vi "Netburner_cntlfull.vi"(0 "Phase Volt":dbl=6.500000000000002 min=-9.0 max=9.0 step=0.0005 format="%_5f", 1 "Tune Volt":dbl=0.3670000000000009 min=-9.9 max=9.9 step=0.0005 format="%_5g", 3 "# Data":i32=80 min=1 max=500 step=1, 5 "IF Atten (dB)":i8=3 min=0 max=31 step=1, 7 "NMR ADC":i32 min=0 max=3 step=1, 8 "Hi Gain":bool, 9 "Tank RF":bool, 11 "LogOff Volt":dbl=-5.996000000000003 min=0.0 max=9.0 step=0.0005 format="%_5f", 12 "IFOff Volt":dbl=5.450461000000012 min=-9.9 max=9.9 step=0.0005 format="%_4g", 14 "# f steps":i32=81 min=1 max=1000 step=1) -> (2 "Temp (C)":dbl=26.88 format="%#_5g", 4 "ADC value":dbl[](array[numeric])=[-0.0314, -0.0313, -0.0297, -0.0295, -0.0285, -0.0272, -0.026, -0.0257, -0.0236, -0.0229, -0.0227, -0.0232, -0.0213, -0.0193, -0.0187, -0.018, -0.0166, -0.0148, -0.0136, -0.0136, -0.0124, -0.0123, -0.0121, -0.0127, -0.0131, -0.0123, -0.0127, -0.0125, -0.0133, -0.0128, -0.0117, -0.012, -0.0128, -0.0138, -0.0149, -0.0166, -0.0211, -0.0291, -0.0424, -0.043, -0.0352, -0.0325, -0.0302, -0.0273, -0.0269, -0.0277, -0.026, -0.0263, -0.0242, -0.021, -0.0178, -0.0171, -0.0172, -0.0168, -0.0161, -0.0168, -0.0178, -0.0197, -0.0204, -0.0197, -0.0175, -0.0187, -0.0188, -0.0202, -0.0207, -0.0229, -0.0238, -0.0251, -0.0264, -0.0268, -0.0278, -0.0301, -0.0313, -0.0334, -0.0364, -0.0377, -0.0382, -0.0394, -0.043, -0.0442, -0.0438], 6 "ADC Std Dev":dbl=0.0009679012345679012 format="%#_4g", 10 "Max ADC":dbl=-0.0117 format="%#_5g", 13 "Volts":dbl=3.245 format="%#_5g", 15 "Min ADC":dbl=-0.0442 format="%#_5g")   [LabVIEW 2013]
uses:
  Global 2.vi
  <vilib>/Analysis/NI_AALBase.lvlib
panel:
  in  "First":bool=TRUE
  out "Begin string":string
  out "ADC Voltage Chart":dbl(graph)=-0.0438
  out "Mean ADC":dbl=-0.023260493827160496 format="%#_5g"
  out "ADC result string":string=" 6.5000  0.3670 -5.9960  5.4505 0 80 81 6 0 0\r26.88  3.245  \r\n-0.0314 0.0005  \r\n-0.0313 0.0007  \r\n-0.0297 0.0008  \r\n-0.0295 0.0007  \r\n-0.0285 0.0009  \r\n-0.0272 0.0007  \r\n-0.0260 0.0009  \r\n-0.0257 0.0007  \r\n-0.0236 0.0008  \r\n-0.0229 0.0008  \r\n-0.0227 0.0009  \r\n-0.0232 0.0011  \r\n-0.0213 0.0010  \r\n-0.0193 0.0014  \r\n-0.0187 0.0009  \r\n-0.0180 0.0007  \r\n-0.0166 0.0010  \r\n-0.0148 0.0006  \r\n-0.0136 0.0007  \r\n-0.0136 0.0010  \r\n-0.0124 0.0006  \r\n-0.0123 0.0007  \r\n-0.0121 0.0007  \r\n-0.0127 0.0006  \r\n-0.0131 0.0006  \r\n-0.0123 0.0007  \r\n-0.0127 0.0007  \r\n-0.0125 0.0006  \r\n-0.0133 0.0006  \r\n-0.0128 0.0009  \r\n-0.0117 0.0006  \r\n-0.0120 0.0008  \r\n-0.0128 0.0006  \r\n-0.0138 0.0007  \r\n-0.0149 0.0009  \r\n-0.0166 0.0016  \r\n-0.0211 0.0031  \r\n-0.0291 0.0059  \r\n-0.0424 0.0009  \r\n-0.0430 0.0037  \r\n-0.0352 0.0010  \r\n-0.0325 0.0013  \r\n-0.0302 0.0016  \r\n-0.0273 0.0006  \r\n-0.0269 0.0007  \r\n-0.0277 0.0007  \r\n-0.0260 0.0009  \r\n-0.0263 0.0015  \r\n-0.0242 0.0014  \r\n-0.0210 0.0013  \r\n-0.0178 0.0010  \r\n-0.0171 0.0007  \r\n-0.0172 0.0007  \r\n-0.0168 0.0007  \r\n-0.0161 0.0006  \r\n-0.0168 0.0005  \r\n-0.0178 0.0010  \r\n-0.0197 0.0008  \r\n-0.0204 0.0010  \r\n-0.0197 0.0006  \r\n-0.0175 0.0006  \r\n-0.0187 0.0006  \r\n-0.0188 0.0010  \r\n-0.0202 0.0007  \r\n-0.0207 0.0006  \r\n-0.0229 0.0008  \r\n-0.0238 0.0009  \r\n-0.0251 0.0009  \r\n-0.0264 0.0008  \r\n-0.0268 0.0009  \r\n-0.0278 0.0008  \r\n-0.0301 0.0007  \r\n-0.0313 0.0006  \r\n-0.0334 0.0012  \r\n-0.0364 0.0009  \r\n-0.0377 0.0006  \r\n-0.0382 0.0007  \r\n-0.0394 0.0013  \r\n-0.0430 0.0012  \r\n-0.0442 0.0008  \r\n-0.0438 0.0009  \r\n?\r\n"
  out "#  Data Bytes Read":u32=1523
  out "DAC, ADC String":string=" 6.5000  0.3670 -5.9960  5.4505 0 80 81 6 0 0"
  out "Error Out":errorcluster={"status"=FALSE, "code"=1073676294, "source"="VISA Read in Netburner_RD.vi->Netburner_cntl6.vi"}
  in  "Error In (none)":errorcluster
  out "COM Port #":refnum<visa-resource-name>="COM9"
  # "Netburner ADC/DAC Test Interface"
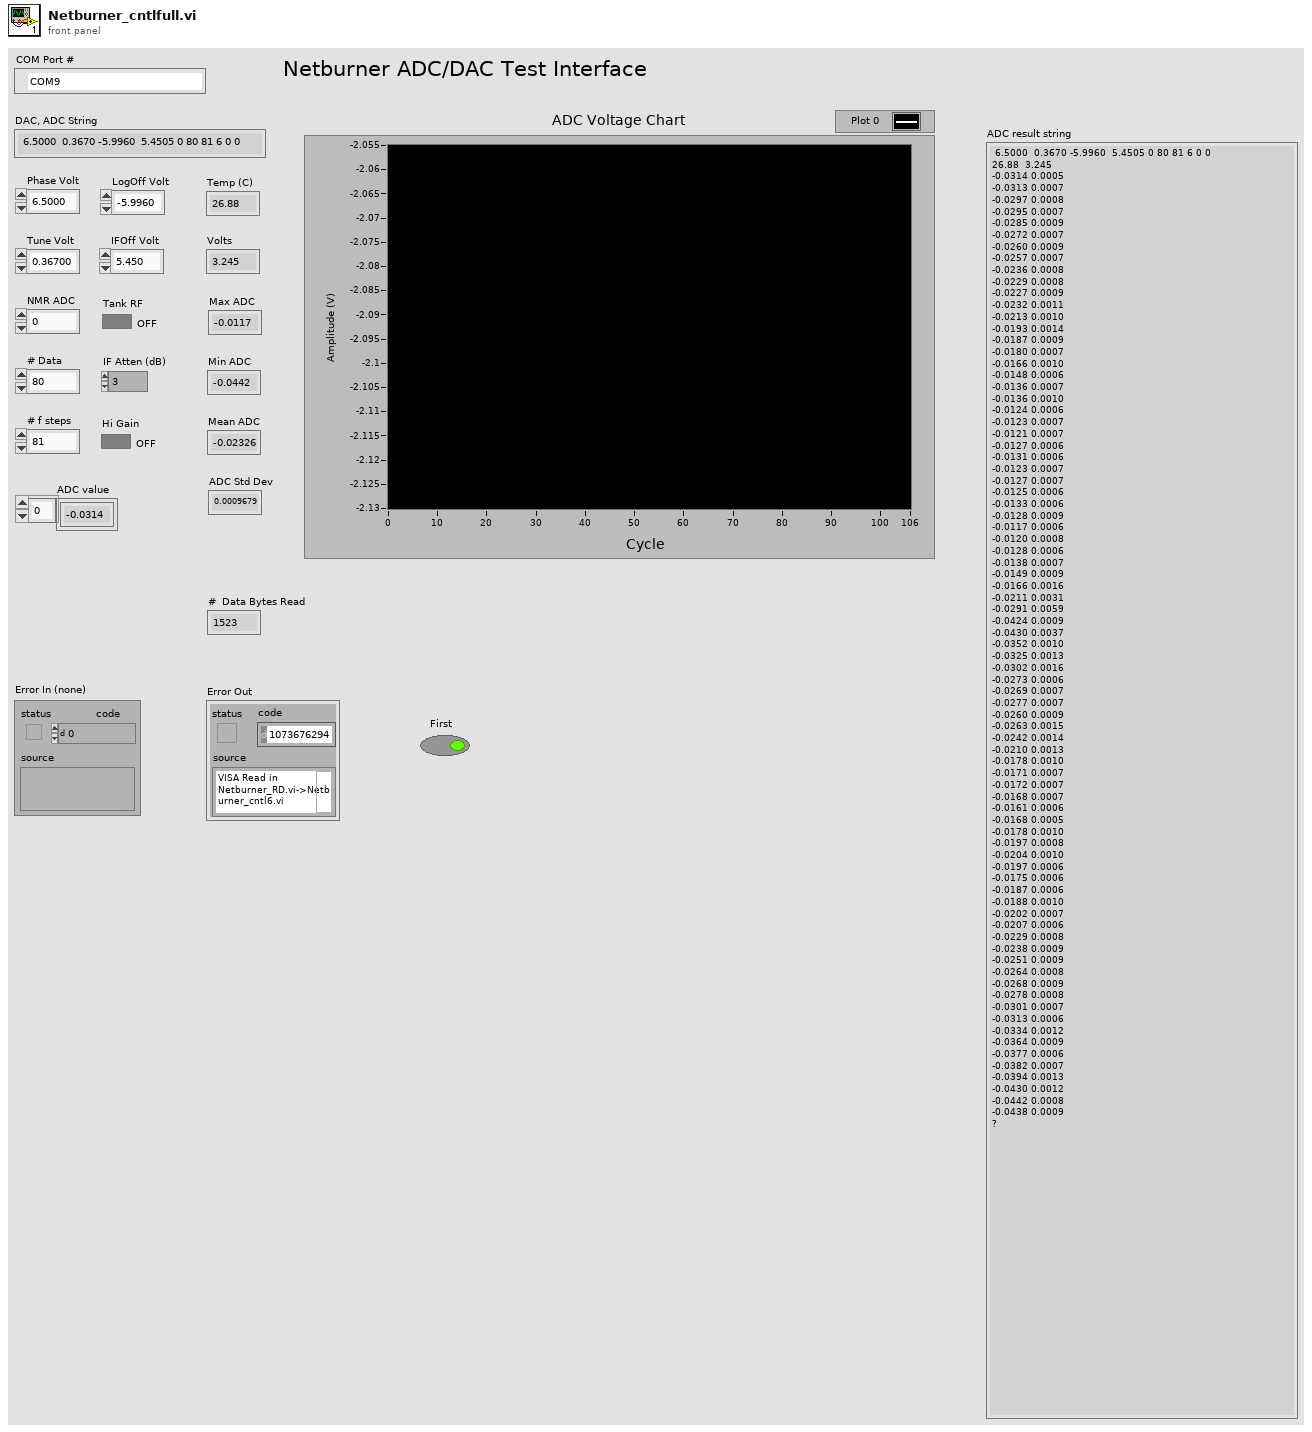
[diagram p1: front panel]
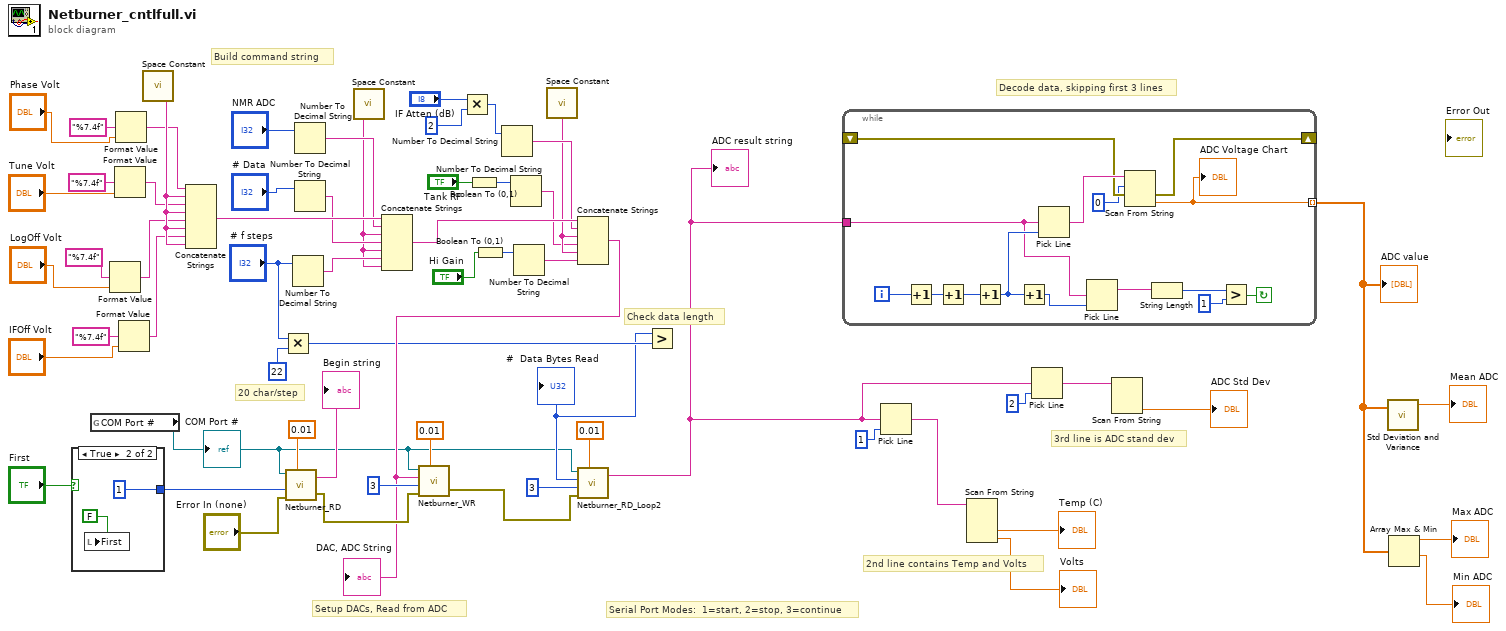
[diagram p0: block diagram]
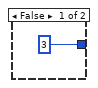
[diagram p2: hidden frame]
diagram:
  # "3rd line is ADC stand dev"
  # "20 char/step"
  # "Check data length"
  # "2nd line contains Temp and Volts"
  # "Build command string"
  # "Decode data, skipping first 3 lines"
  # "Serial Port Modes:  1=start, 2=stop, 3=continue"
  # "Setup DACs, Read from ADC"
  n1 = case shown="True" "First" {
    tunnel: [3 1] -> w6
    frame False {
    }
    frame True {
      n2 = local write "First"(FALSE) -> ()
    }
  }
  n3 = global read "Global 2.vi" "COM Port #"() -> (w5:refnum<visa-resource-name>)
  "COM Port #" <- w5
  n4 = Format Value(format string="%7.4f", value (0)="LogOff Volt") -> (output string=w8:string)  [unwired: 1 in]
  n5 = Format Value(format string="%7.4f", value (0)="Tune Volt") -> (output string=w38:string)  [unwired: 1 in]
  n6 = Format Value(format string="%7.4f", value (0)="Phase Volt") -> (output string=w10:string)  [unwired: 1 in]
  n7 = Format Value(format string="%7.4f", value (0)="IFOff Volt") -> (output string=w41:string)  [unwired: 1 in]
  n8 = call <vilib>:"Space Constant.vi"() -> ("String"=w47:string)
  n9 = Concatenate Strings(w10, w47, w38, w47, w8, w47, w41, w47) -> (w48:string)
  n10 = Multiply(x="# f steps", y=22) -> (x*y=w16:i32)
  n11 = call "Netburner_RD.vi"("VISA resource name (COM Port #)"=w5, "Mode (0)"=w6, "Error In (no error)"="Error In (none)", "Wait (sec)"=0.01) -> ("Return String from Device"=→"Begin string":string, "Error Out"=w60:errorcluster)  [unwired: 1 out]
  n12 = Number To Decimal String(number="# f steps") -> (decimal integer string=w44:string)  [unwired: 1 in]
  n13 = Number To Decimal String(number="NMR ADC") -> (decimal integer string=w46:string)  [unwired: 1 in]
  n14 = Number To Decimal String(number="# Data") -> (decimal integer string=w45:string)  [unwired: 1 in]
  n15 = call <vilib>:"Space Constant.vi"() -> ("String"=w35:string)
  n16 = Concatenate Strings(w48, w46, w35, w45, w35, w44, w35) -> (w37:string)
  n17 = Multiply(x="IF Atten (dB)", y=2) -> (x*y=w24:i32)
  n18 = Boolean To (0,1)(Boolean="Tank RF") -> (0, 1=w32:i16)
  n19 = Boolean To (0,1)(Boolean="Hi Gain") -> (0, 1=w31:i16)
  n20 = Number To Decimal String(number=w24) -> (decimal integer string=w34:string)  [unwired: 1 in]
  n21 = Number To Decimal String(number=w32) -> (decimal integer string=w30:string)  [unwired: 1 in]
  n22 = Number To Decimal String(number=w31) -> (decimal integer string=w29:string)  [unwired: 1 in]
  n23 = call <vilib>:"Space Constant.vi"() -> ("String"=w33:string)
  n24 = Concatenate Strings(w37, w34, w33, w30, w33, w29) -> (w36:string)
  "DAC, ADC String" <- w36
  n25 = call "Netburner_WR.vi"("VISA resource name (COM Port #)"=w5, "String to Send"=w36, "Mode (0)"=3, "Error In (no error)"=w60, "Wait (sec)"=0.01) -> ("Error Out"=w56:errorcluster)  [unwired: 1 in]
  n26 = call "Netburner_RD_Loop2.vi"("VISA resource name (COM Port #)"=w5, "Mode (0)"=3, "Error In (no error)"=w56, "Wait (sec)"=0.01) -> ("#  Bytes Read"=w15:u32, "Return String from Device"=w3:string)  [unwired: 1 out]
  "#  Data Bytes Read" <- w15
  "ADC result string" <- w3
  n27 = Greater?(x=w15, y=w16) -> ()  [unwired: 1 out]
  n28 = while {
    tunnel: w3 -> [w76]
    tunnel: [w74] -> w53 mode=indexing
    shift-right: [w68] -> _
    shift-left: _ -> [w69]
    i -> [w65]
    stop <- w73 continue-if-true
    n29 = Increment(x=w65) -> (x+1=w66:i32)
    n30 = Increment(x=w66) -> (x+1=w70:i32)
    n31 = Increment(x=w70) -> (x+1=w78:i32)
    n32 = Increment(x=w78) -> (x+1=w77:i32)
    n33 = Pick Line(multi-line string=w76, line index=w78) -> (output string=w79:string)  [unwired: 1 in]
    n34 = Pick Line(multi-line string=w76, line index=w77) -> (output string=w75:string)  [unwired: 1 in]
    n35 = Scan From String "Scan From String"(input string=w79, initial scan location=0, error in=w69) -> (error out=w68:errorcluster, output 1=w74:dbl)  [unwired: 2 in, 2 out]
    "ADC Voltage Chart" <- w74
    n36 = String Length(string=w75) -> (length=w72:i32)
    n37 = Greater?(x=w72, y=1) -> (0:w73:bool)
  }
  "ADC value" <- w53
  n38 = Pick Line(multi-line string=w3, line index=1) -> (output string=w22:string)  [unwired: 1 in]
  n39 = Scan From String "Scan From String"(input string=w22) -> (output 1=→"Temp (C)":dbl, output 2=→"Volts":dbl)  [unwired: 5 in, 3 out]
  n40 = Pick Line(multi-line string=w3, line index=2) -> (output string=w2:string)  [unwired: 1 in]
  n41 = Scan From String "Scan From String"(input string=w2) -> (output 1=→"ADC Std Dev":dbl)  [unwired: 4 in, 3 out]
  n42 = call <vilib>:"Std Deviation and Variance.vi"("X"=w53) -> ("mean"=→"Mean ADC":dbl)  [unwired: 1 in, 2 out]
  n43 = Array Max & Min(array=w53) -> (max value=→"Max ADC":dbl, min value=→"Min ADC":dbl)  [unwired: 2 out]
